vi "Zip.vi"() -> ()   [LabVIEW 2018]
panel:
  in  "Local file name":path=path "CuspControl_RT.zip"
  # "LabVIEW .zip subvi's error out if I try to automate delete-overwrite\nso just make sure the file does not already exist\nbefore running this VI"
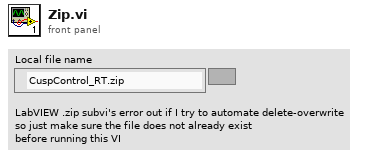
[diagram p1: front panel]
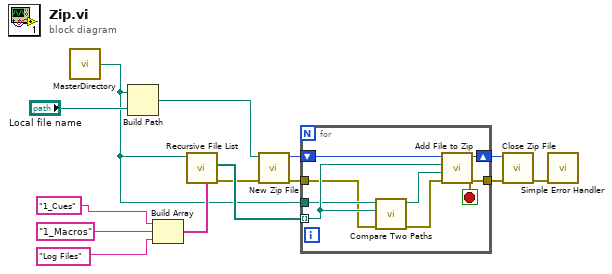
[diagram p0: block diagram]
diagram:
  n1 = call "MasterDirectory.vi"() -> ("Master Directory"=w2:path)
  n2 = Build Path(base path=w2, name or relative path="Local file name") -> (appended path=w1:path)
  n3 = Build Array("1_Cues", "1_Macros", "Log Files") -> (w11:string[])
  n4 = call <vilib>:"Recursive File List.vi"("Folders to Exclude"=w11, "Folder Path"=w2) -> ("error out"=w8:errorcluster, "All Files in Dir"=w9:path[])  [unwired: 5 in, 3 out]
  n5 = call <vilib>:"New Zip File.vi"("error in (no error)"=w8, "target"=w1) -> ("error out"=w5:errorcluster, "zip file out"=w4:i64)  [unwired: 1 in, 3 out]
  n6 = for {
    tunnel: w9 -> [w19] mode=indexing
    tunnel: w5 -> [w16]
    tunnel: [w20] -> w6
    shift-right: [w21] -> w7
    shift-left: w4 -> [w22]
    tunnel: w2 -> [w18]
    stop <- w20 stop-if-true
    n7 = call <vilib>:"Compare Two Paths.vi"("error in (no error)"=w16, "Path 2"=w19, "Path 1"=w18) -> ("error out"=w15:errorcluster, "Relative Path from 1 to 2"=w17:path)  [unwired: 5 in, 2 out]
    n8 = call <vilib>:"Add File to Zip.vi"("error in (no error)"=w15, "destination path in zip"=w17, "source file path"=w19, "zip file in"=w22) -> ("error out"=w20:errorcluster, "zip file out"=w21:i64)  [unwired: 6 out]
  }
  n9 = call <vilib>:"Close Zip File.vi"("error in (no error)"=w6, "zip file in"=w7) -> ("error out"=w3:errorcluster)  [unwired: 1 in, 4 out]
  n10 = call <vilib>:"Simple Error Handler.vi"("error in (no error)"=w3) -> ()  [unwired: 1 in, 8 out]
